vi "motors_move_axis.vi"(8 "Error In":errorcluster, 9 "Position":u16, 10 "Axis":T1, 11 "VISA resource name":refnum<visa-resource-name>) -> (0 "Error Out":errorcluster, 3 "VISA resource name out":refnum<visa-resource-name>)   [LabVIEW 2019]
uses:
  motors_axis_enum_typedef.ctl
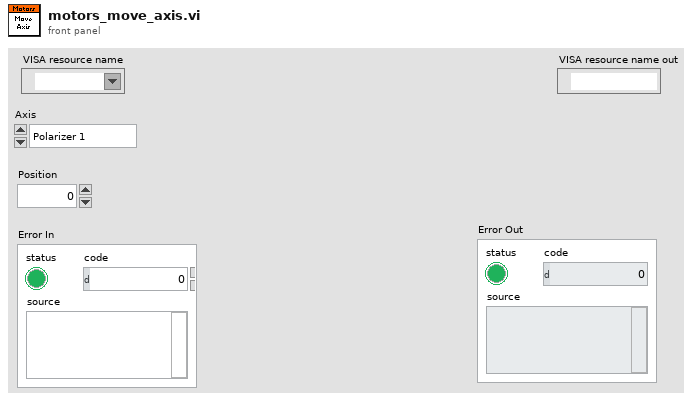
[diagram p1: front panel]
types:
  T1 = typedef "motors_axis_enum_typedef.ctl" = enum16{"Polarizer 1", "Polarizer 2", "Sample", "Stage"}
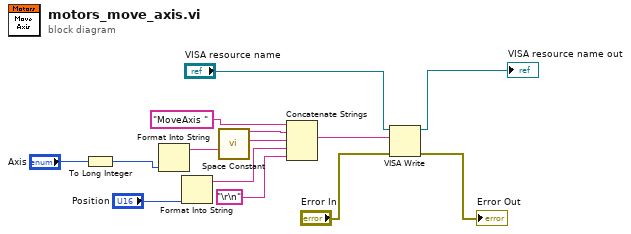
[diagram p0: block diagram]
diagram:
  n1 = To Long Integer(number="Axis") -> (32bit integer=w2:i32)
  n2 = Format Into String(w2) -> (resulting string=w1:string)  [unwired: 3 in, 1 out]
  n3 = Format Into String("Position") -> (resulting string=w10:string)  [unwired: 3 in, 1 out]
  n4 = call <vilib>:"Space Constant.vi"() -> ("String"=w11:string)
  n5 = Concatenate Strings("MoveAxis ", w1, w11, w10, "\r\n") -> (w7:string)
  n6 = VISA Write(VISA resource name="VISA resource name", write buffer=w7, error in (no error)="Error In") -> (VISA resource name out=→"VISA resource name out":refnum<visa-resource-name>, error out=→"Error Out":errorcluster)  [unwired: 1 out]
